vi "Calculate Chunk string size.vi"(0 "String":string, 5 "Font":T2={"Name"="", "Size"=12.0, "Color"=0, "Style"={"Bold"=FALSE, "Italic"=FALSE, "Underline"=FALSE, "Strikeout"=FALSE}, "Type"={"Type&direction"=enum."Select", "Embedded"=FALSE, "Encoding"=""}}, 7 "Font refnum":refnum<k24>, 9 "System Fonts":T1, 11 "error in (no error)":errorcluster) -> (4 "DescentPoint":sgl, 6 "Width":sgl, 10 "Height":sgl, 15 "error out":errorcluster)   [LabVIEW 2019]
doc: "Version 1.0\nDeveloped by Jean-Marc Simard\nCopyright © 2010, Exaprom Inc.\nAll rights reserved.\nLicense: BSD\n\nWith iTextSharp 4.1.6 (http://itextsharp.sourceforge.net)\nunder Mozilla Public License Version 1.1\n(http://www.mozilla.org/MPL/MPL-1.1.html)"
uses:
  <userlib>/Exaprom PDF/Controls/Font Controls/Font complete cluster.ctl
  <userlib>/Exaprom PDF/Controls/Font Controls/Font size.ctl
  <userlib>/Exaprom PDF/Controls/Font Controls/Font color.ctl
  <userlib>/Exaprom PDF/Controls/Font Controls/Type and encoding.ctl
  <userlib>/Exaprom PDF/Controls/Text Controls/Unicode/Type and run direction.ctl
  <userlib>/Exaprom PDF/Controls/Font Controls/System Fonts.ctl
  C:/Program Files/National Instruments/LabVIEW 2019/user.lib/Exaprom PDF/DLL/itextsharp.dll
  DLL/itextsharp.dll
  <userlib>/Exaprom PDF/LV Class/Fonts Class/Font Class.lvclass
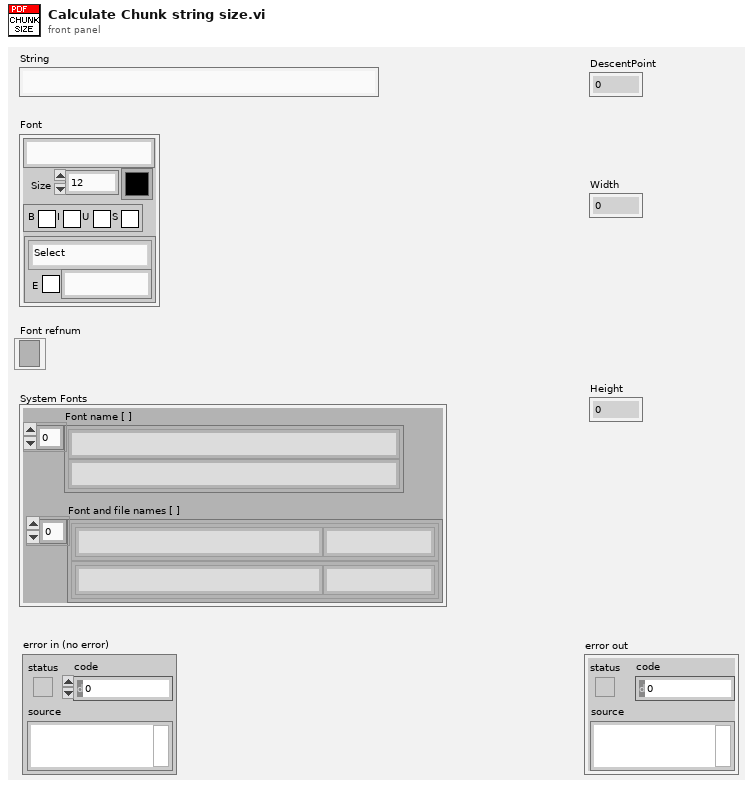
[diagram p1: front panel]
types:
  T1 = typedef "System Fonts.ctl" = cluster{"Font name [ ]":string[], "Font and file names [ ]":cluster{"Font name":string, "File name":string}[]}
  T2 = typedef "Font complete cluster.ctl" = cluster{"Name":string, "Size":T3, "Color":T4, "Style":cluster{"Bold":bool, "Italic":bool, "Underline":bool, "Strikeout":bool}, "Type":T5}
  T3 = typedef "Font size.ctl" = sgl
  T4 = typedef "Font color.ctl" = u32
  T5 = typedef "Type and encoding.ctl" = cluster{"Type&direction":T6, "Embedded":bool, "Encoding":string}
  T6 = typedef "Type and run direction.ctl" = enum16{"Select", "ASCII", "UTF-16", "UTF-16 (default)", "UTF-16 (LTR)", "UTF-16 (RTL)"}
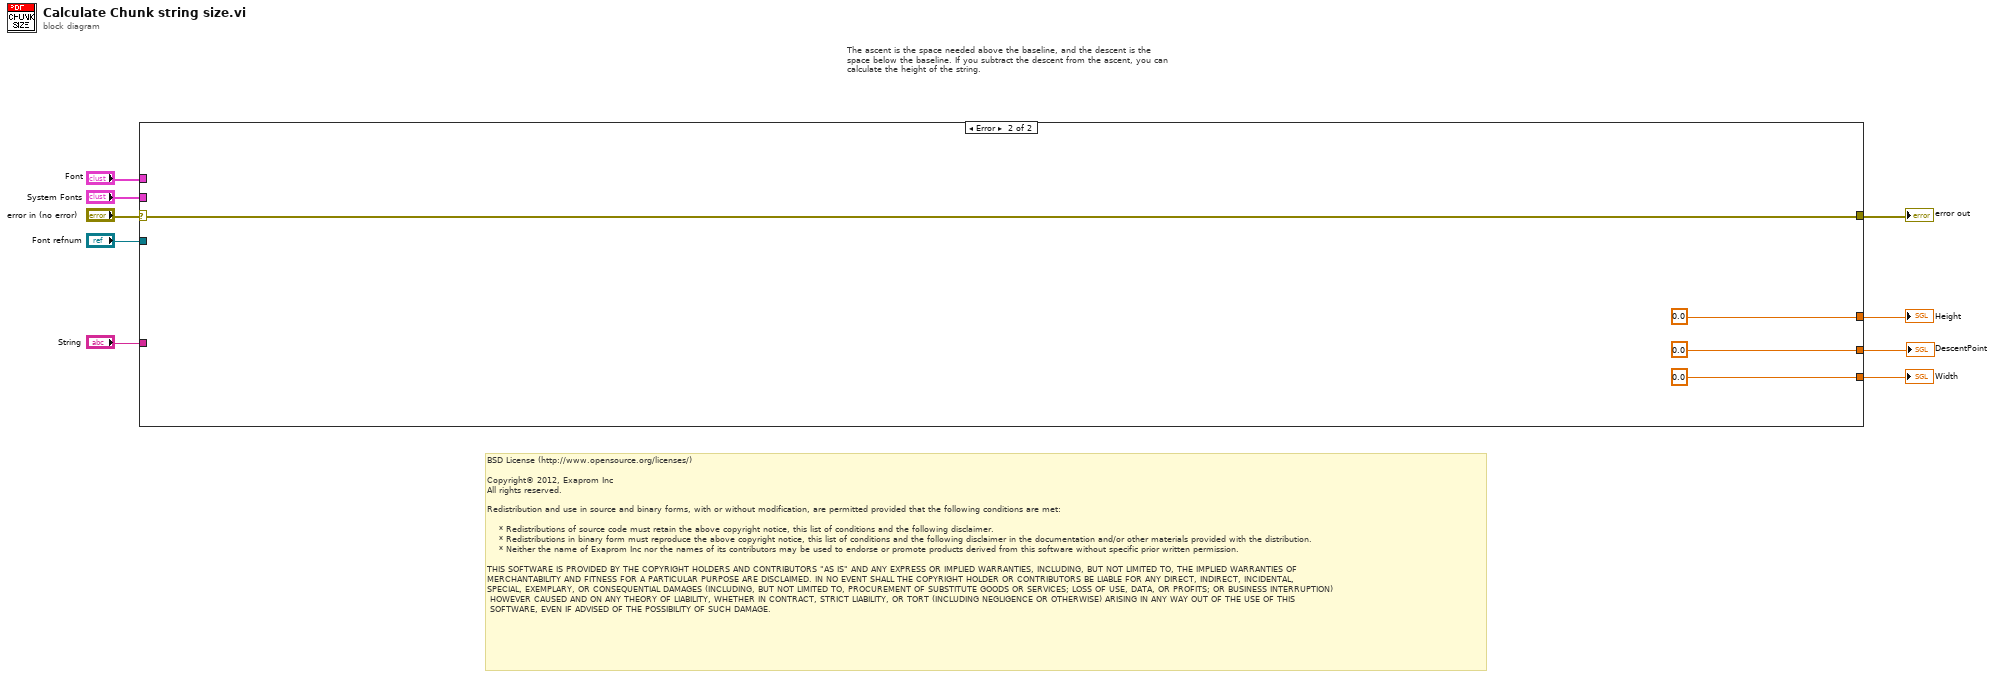
[diagram p0: block diagram]
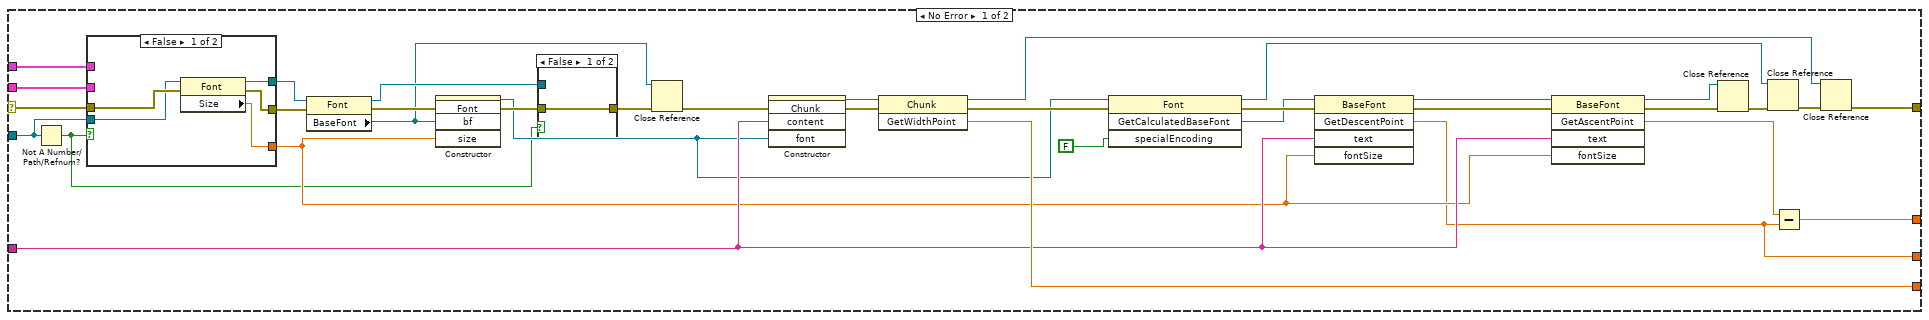
[diagram p2: hidden frame]
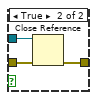
[diagram p3: hidden frame]
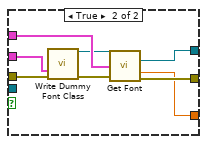
[diagram p4: hidden frame]
diagram:
  # "The ascent is the space needed above the baseline, and the descent is the\nspace below the baseline. If you subtract the descent from the ascent, you can\ncalculate the height of the string."
  # "BSD License (http://www.opensource.org/licenses/)\n\nCopyright© 2012, Exaprom Inc\nAll rights reserved.\n\nRedistribution and use in source and binary forms, with or without modification, are permitted provided that the following conditions are met:\n\n    * Redistributions of source code must retain the above copyright notice, this list of conditions and the following disclaimer.\n    * Redistributions in binary form must reproduce the above copyright notice, this list of conditions and the following disclaimer in the documentation and/or other materials provided with the distribution.\n    * Neither the name of Exaprom Inc nor the names of its contributors may be used to endorse or promote products derived from this software without specific prior written permission.\n\nTHIS SOFTWARE IS PROVIDED BY THE COPYRIGHT HOLDERS AND CONTRIBUTORS \"AS IS\" AND ANY EXPRESS OR IMPLIED WARRANTIES, INCLUDING, BUT NOT LIMITED TO, THE IMPLIED WARRANTIES OF \nMERCHANTABILITY AND FITNESS FOR A PARTICULAR PURPOSE ARE DISCLAIMED. IN NO EVENT SHALL THE COPYRIGHT HOLDER OR CONTRIBUTORS BE LIABLE FOR ANY DIRECT, INDIRECT, INCIDENTAL,\nSPECIAL, EXEMPLARY, OR CONSEQUENTIAL DAMAGES (INCLUDING, BUT NOT LIMITED TO, PROCUREMENT OF SUBSTITUTE GOODS OR SERVICES; LOSS OF USE, DATA, OR PROFITS; OR BUSINESS INTERRUPTION)\n HOWEVER CAUSED AND ON ANY THEORY OF LIABILITY, WHETHER IN CONTRACT, STRICT LIABILITY, OR TORT (INCLUDING NEGLIGENCE OR OTHERWISE) ARISING IN ANY WAY OUT OF THE USE OF THIS\n SOFTWARE, EVEN IF ADVISED OF THE POSSIBILITY OF SUCH DAMAGE."
  n1 = case shown="Error" "error in (no error)" {
    selector: "error in (no error)" -> [w24 w65]
    tunnel: [w41 sgl 0.0 ("GetWidthPoint")] -> w9
    tunnel: [w40 sgl 0.0] -> w8
    tunnel: "String" -> [w31 _]
    tunnel: [w30 w65] -> w6
    tunnel: "Font" -> [w26 _]
    tunnel: [w22 sgl 0.0 ("GetDescentPoint")] -> w3
    tunnel: "System Fonts" -> [w23 _]
    tunnel: "Font refnum" -> [w13 _]
    frame No Error {
      n2 = Not A Number/Path/Refnum?(number/path/refnum=w13) -> (NaN/Path/Refnum?=w12:bool)
      n3 = case shown="False" w12 {
        tunnel: [w49 w61] -> w29
        tunnel: [w51 w60] -> w28
        tunnel: [w50 w59] -> w27
        tunnel: w26 -> [_ w58]
        tunnel: w24 -> [w53 w57]
        tunnel: w23 -> [_ w55]
        tunnel: w13 -> [w52 _]
        frame False {
          n4 = property class="Font"(reference=w52, error in=w53) -> (reference out=w49:refnum<k24>, error out=w51:errorcluster, "Size"=w50:sgl)
        }
        frame True {
          n5 = call <userlib>:"Write Dummy Font Class.vi"("System Fonts"=w55, "error in (no error)"=w57) -> ("Font OUT"=w54:refnum<class "Font Class.lvclass">, "error out"=w56:errorcluster)  [unwired: 12 in]
          n6 = call <userlib>:"Get Font.vi"("Font"=w54, "Font IN"=w58, "error in (no error)"=w56) -> ("Font"=w61:refnum<k24>, "Font Size"=w59:T3, "error out"=w60:errorcluster)  [unwired: 8 in, 2 out]
        }
      }
      n7 = property class="Font"(reference=w29, error in=w28) -> (reference out=w21:refnum<k24>, error out=w20:errorcluster, "BaseFont"=w16:refnum<k24>)
      n8 = constructor class="Font"(error in=w20, "bf"=w16, "size"=w27) -> (reference out=w15:refnum<k24>, error out=w19:errorcluster)  [unwired: 2 in, 3 out]
      n9 = case shown="False" w12 {
        tunnel: w21 -> [_ w48]
        tunnel: w19 -> [w45 w47]
        tunnel: [w45 w46] -> w18
        frame False {
        }
        frame True {
          n10 = Close Reference(reference=w48, error in (no error)=w47) -> (error out=w46:errorcluster)
        }
      }
      n11 = Close Reference(reference=w16, error in (no error)=w18) -> (error out=w17:errorcluster)
      n12 = constructor class="Chunk"(error in=w17, "content"=w31, "font"=w15) -> (reference out=w11:refnum<k24>, error out=w10:errorcluster)  [unwired: 2 in, 3 out]
      n13 = invoke class="Chunk" method="GetWidthPoint"(reference=w11, error in=w10) -> (reference out=w32:refnum<k24>, error out=w37:errorcluster, "GetWidthPoint"=w41:sgl)  [unwired: 1 in]
      n14 = invoke class="Font" method="GetCalculatedBaseFont"(reference=w15, error in=w37, "specialEncoding"=FALSE) -> (reference out=w34:refnum<k24>, error out=w39:errorcluster, "GetCalculatedBaseFont"=w25:refnum<k24>)  [unwired: 1 in, 1 out]
      n15 = invoke class="BaseFont" method="GetDescentPoint"(reference=w25, error in=w39, "text"=w31, "fontSize"=w27) -> (reference out=w43:refnum<k24>, error out=w42:errorcluster, "GetDescentPoint"=w22:sgl)  [unwired: 1 in, 2 out]
      n16 = invoke class="BaseFont" method="GetAscentPoint"(reference=w43, error in=w42, "text"=w31, "fontSize"=w27) -> (reference out=w14:refnum<k24>, error out=w36:errorcluster, "GetAscentPoint"=w38:sgl)  [unwired: 1 in, 2 out]
      n17 = Close Reference(reference=w14, error in (no error)=w36) -> (error out=w35:errorcluster)
      n18 = Close Reference(reference=w34, error in (no error)=w35) -> (error out=w33:errorcluster)
      n19 = Subtract(x=w38, y=w22) -> (x-y=w40:sgl)
      n20 = Close Reference(reference=w32, error in (no error)=w33) -> (error out=w30:errorcluster)
    }
    frame Error {
    }
  }
  "Width" <- w9
  "Height" <- w8
  "error out" <- w6
  "DescentPoint" <- w3
